vi "Example Input.vi"() -> ()   [LabVIEW 2010]
uses:
  C:/tf/play/labview/Tinkerforge.dll
  Tinkerforge.dll
panel:
  out "value":bool[](array[boolean])
  in  "uid":string="cnq"
  in  "port":i32=4223
  in  "host":string="localhost"
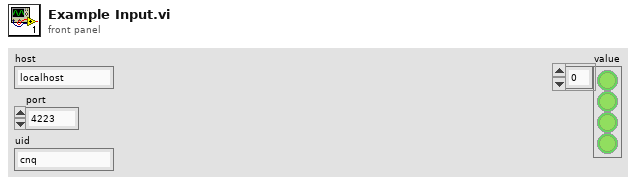
[diagram p1: front panel]
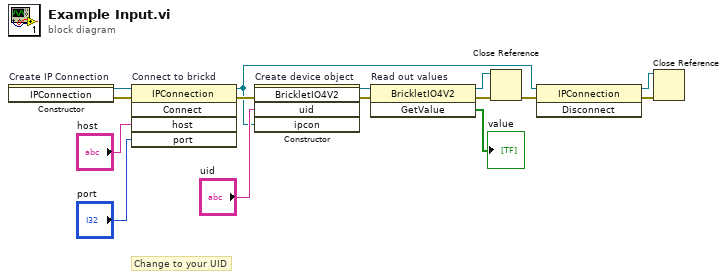
[diagram p0: block diagram]
diagram:
  # "Change to your UID"
  n1 = constructor on="Create IP Connection" class="IPConnection"() -> (reference out=w15:refnum<k24>, error out=w3:errorcluster)  [unwired: 3 in, 1 out]
  n2 = invoke on="Connect to brickd" class="IPConnection" method="Connect"(reference=w15, error in=w3, "host"="host", "port"="port") -> (reference out=w5:refnum<k24>, error out=w11:errorcluster)  [unwired: 1 in, 3 out]
  n3 = constructor on="Create device object" class="BrickletIO4V2"(error in=w11, "uid"="uid", "ipcon"=w5) -> (reference out=w10:refnum<k24>, error out=w2:errorcluster)  [unwired: 2 in, 3 out]
  n4 = invoke on="Read out values" class="BrickletIO4V2" method="GetValue"(reference=w10, error in=w2) -> (reference out=w8:refnum<k24>, error out=w9:errorcluster, "GetValue"=→"value":bool[])  [unwired: 1 in]
  n5 = Close Reference(reference=w8, error in (no error)=w9) -> (error out=w7:errorcluster)
  n6 = invoke class="IPConnection" method="Disconnect"(reference=w5, error in=w7) -> (reference out=w4:refnum<k24>, error out=w6:errorcluster)  [unwired: 1 in, 1 out]
  n7 = Close Reference(reference=w4, error in (no error)=w6) -> ()  [unwired: 1 out]
